vi "SCE_Draw Flattened Pixmap.vi"(8 "image data":T1, 9 "picture":picture) -> (3 "new picture":picture)   [LabVIEW 2018]
doc: "Draws a 1-, 4-, or 8-bit pixmap or a 24-bit RGB pixmap into a picture."
uses:
  <vilib>/picture/picture.llb/imagedata.ctl
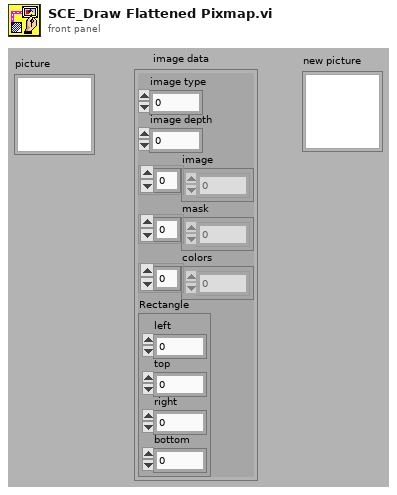
[diagram p1: front panel]
types:
  T1 = typedef "imagedata.ctl" = cluster{"image type":i32, "image depth":i32, "image":u8[], "mask":u8[], "colors":u32[], "Rectangle":cluster{"left":i16, "top":i16, "right":i16, "bottom":i16}}
  T2 = cluster{"default foreground":u32, "default background":u32}
  T3 = cluster{"left":i16, "top":i16, "right":i16, "bottom":i16}
  T4 = cluster{"top":i16, "left":i16, "bottom":i16, "right":i16}
  T5 = cluster{"opcode-Copy Pixmap":i16, i32, i32, cluster{"top":i16, "left":i16, "bottom":i16, "right":i16}, i16, "output cluster":cluster{"default foreground":u32, "default background":u32}}
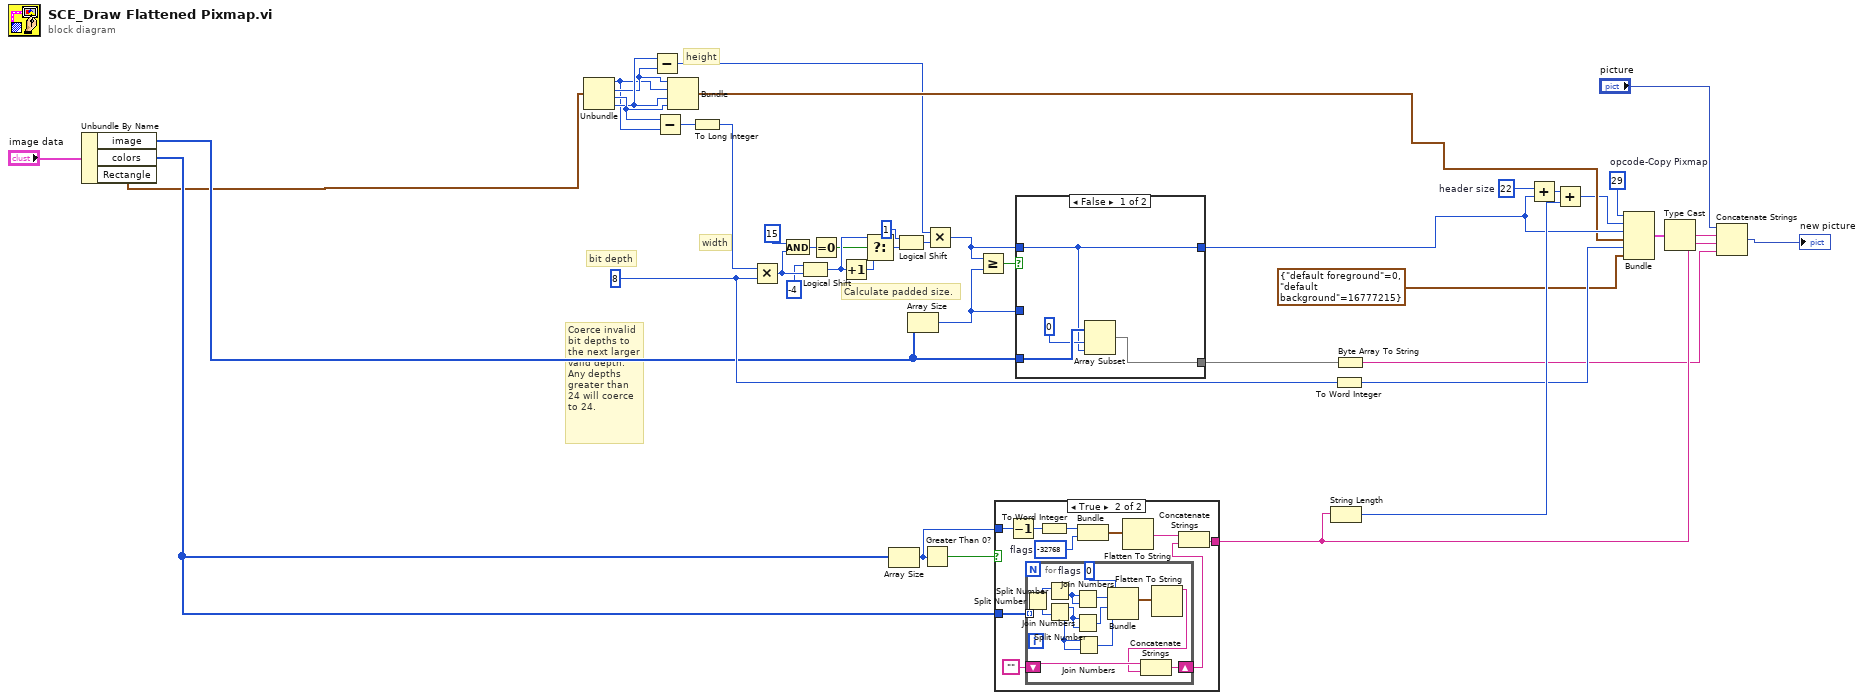
[diagram p0: block diagram]
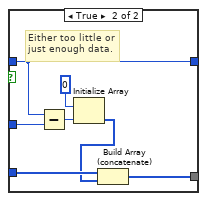
[diagram p2: hidden frame]
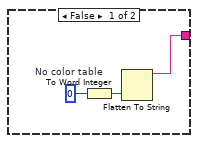
[diagram p3: hidden frame]
diagram:
  w29 = 8
  w15 = i16 22  # header size
  w13 = i16 29  # opcode-Copy Pixmap
  # "Calculate padded size."
  # "Coerce invalid\nbit depths to\nthe next larger\nvalid depth.\nAny depths\ngreater than\n24 will coerce\nto 24."
  # "bit depth"
  # "height"
  # "width"
  n1 = Unbundle By Name("image data") -> ("image"=w19:u8[], "colors"=w24:u32[], "Rectangle"=w12:T3)
  n2 = Unbundle(w12) -> ("left"=w21:i16, "top"=w36:i16, "right"=w38:i16, "bottom"=w37:i16)
  n3 = Subtract(x=w37, y=w36) -> (x-y=w22:i16)
  n4 = Subtract(x=w38, y=w21) -> (x-y=w28:i16)
  n5 = Bundle("top"=w36, "left"=w21, "bottom"=w37, "right"=w38) -> (w23:T4)  [unwired: 1 in]
  n6 = To Long Integer(number=w28) -> (32bit integer=w20:i32)
  n7 = Multiply(x=w20, y=w29) -> (x*y=w3:i32)
  n8 = And(x=15, y=w3) -> (x .and. y?=w5:i32)
  n9 = Logical Shift(y=-4, x=w3) -> (x << y=w7:i32)
  n10 = Equal To 0?(x=w5) -> (x = 0?=w6:bool)
  n11 = Increment(x=w7) -> (x+1=w8:i32)
  n12 = Select(t=w7, s=w6, f=w8) -> (s? t:f=w10:i32)
  n13 = Array Size(array=w24) -> (size(s)=w43:i32)
  n14 = Logical Shift(y=1, x=w10) -> (x << y=w11:i32)
  n15 = Array Size(array=w19) -> (size(s)=w32:i32)
  n16 = Greater Than 0?(x=w43) -> (x > 0?=w30:bool)
  n17 = Multiply(x=w22, y=w11) -> (x*y=w34:i32)
  n18 = Greater Or Equal?(x=w34, y=w32) -> (x >= y?=w35:bool)
  n19 = case shown="True" w30 {
    tunnel: w24 -> [_ w47]
    tunnel: w43 -> [_ w56]
    tunnel: [w44 w51] -> w40
    frame False {
      w46 = 0  # No color table
      n20 = To Word Integer(number=w46) -> (16bit integer=w45:i16)
      n21 = Flatten To String(anything=w45) -> (data string=w44:string)  [unwired: 3 in, 2 out]
    }
    frame True {
      w54 = i16 -32768  # flags
      n22 = Decrement(x=w56) -> (x-1=w48:i32)
      n23 = for {
        tunnel: w47 -> [w68] mode=indexing
        shift-right: [w65] -> w49
        shift-left: "" -> [w66]
        w67 = i16 0  # flags
        n24 = Split Number(x=w68) -> (hi(x)=w70:u16, lo(x)=w69:u16)
        n25 = Split Number(x=w70) -> (lo(x)=w57:u8)  [unwired: 1 out]
        n26 = Split Number(x=w69) -> (hi(x)=w63:u8, lo(x)=w62:u8)
        n27 = Join Numbers(hi=w57, lo=w57) -> ((hi.lo)=w64:u16)
        n28 = Join Numbers(hi=w63, lo=w63) -> ((hi.lo)=w61:u16)
        n29 = Join Numbers(hi=w62, lo=w62) -> ((hi.lo)=w60:u16)
        n30 = Bundle("flags"=w67, w64, w61, w60) -> (w59:cluster{"flags":i16, u16, u16, u16})  [unwired: 1 in]
        n31 = Flatten To String(anything=w59) -> (data string=w58:string)  [unwired: 3 in, 2 out]
        n32 = Concatenate Strings(w66, w58) -> (w65:string)
      }
      n33 = To Word Integer(number=w48) -> (16bit integer=w55:i16)
      n34 = Bundle(w55, "flags"=w54) -> (w53:cluster{i16, "flags":i16})  [unwired: 1 in]
      n35 = Flatten To String(anything=w53) -> (data string=w52:string)  [unwired: 3 in, 2 out]
      n36 = Concatenate Strings(w52, w49) -> (w51:string)
    }
  }
  n37 = case shown="False" w35 {
    tunnel: w19 -> [w74 w78]
    tunnel: [w73 w79] -> w31
    tunnel: w34 -> [w71 w75]
    tunnel: [w71 w75] -> w33
    tunnel: w32 -> [_ w76]
    frame False {
      n38 = Array Subset(array=w74, index=0, length=w71) -> (w73:u8[])
    }
    frame True {
      # "Either too little or\njust enough data."
      n39 = Subtract(x=w75, y=w76) -> (x-y=w81:i32)
      n40 = Initialize Array(u8 0, w81) -> (w77:u8[])
      n41 = Build Array (concatenate)(w78, w77) -> (w79:u8[])
    }
  }
  n42 = String Length(string=w40) -> (length=w42:i32)
  n43 = To Word Integer(number=w29) -> (16bit integer=w41:i16)
  n44 = Byte Array To String(unsigned byte array=w31) -> (string=w39:string)
  n45 = Add(x=w15, y=w33) -> (x+y=w16:i32)
  n46 = Add(x=w16, y=w42) -> (x+y=w17:i32)
  n47 = Bundle("opcode-Copy Pixmap"=w13, w17, w33, w23, w41, "output cluster"=T2 {"default foreground"=0, "default background"=16777215}) -> (w14:T5)  [unwired: 1 in]
  n48 = Type Cast(x=w14) -> (*(type *) &x=w18:string)  [unwired: 1 in]
  n49 = Concatenate Strings("picture", w18, w40, w39) -> (→"new picture":picture)
